vi "Path as UTF-8 Path (LabVIEW Path).vi"(9 "error in":errorcluster, 10 "Path":path) -> (1 "error out":errorcluster, 2 "UTF-8 Path":refnum<class "UTF-8 Path.lvclass">)   [LabVIEW 2020, in "G-Unicode.lvlib"]
doc: "Converts the input path to a UTF-8 Path. Valid inputs are a UTF-8 Path class, or LabVIEW path."
uses:
  G-Unicode.lvlib
  Types/UTF-8 Path/UTF-8 Path.lvclass
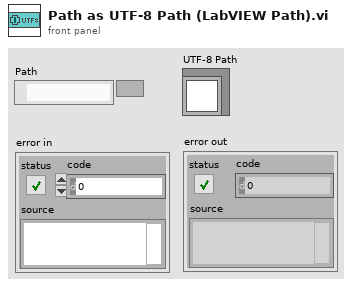
[diagram p1: front panel]
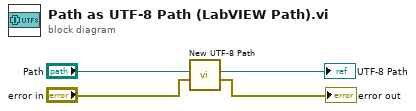
[diagram p0: block diagram]
diagram:
  n1 = call "New UTF-8 Path.vi"("error in"="error in", "LabVIEW Path"="Path") -> ("error out"=→"error out":errorcluster, "UTF-8 Path"=→"UTF-8 Path":refnum<class "UTF-8 Path.lvclass">)  [unwired: 8 in]
